vi "ScaleTo16Bit_IQ_raw.vi"(8 "valid in":bool, 9 "factor":u16, 10 "Q":fxp<+/-,18,1>, 11 "I":fxp<+/-,18,1>) -> (0 "valid out":bool, 3 "32bit integer":u32)   [LabVIEW 2025]
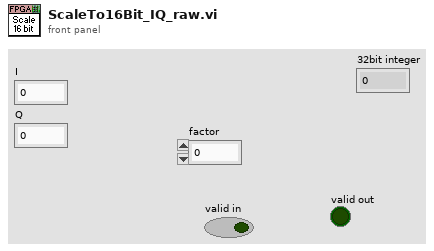
[diagram p1: front panel]
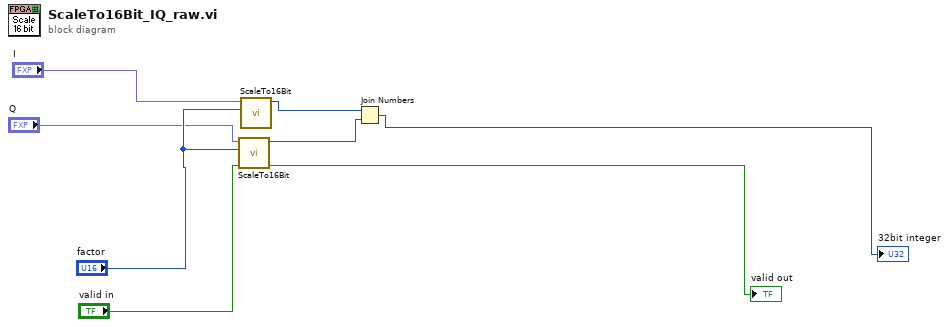
[diagram p0: block diagram]
diagram:
  n1 = call "ScaleTo16Bit.vi"("valid in"="valid in", "factor"="factor", "val"="Q") -> ("valid out"=→"valid out":bool, "16bit integer"=w5:i16)  [unwired: 7 in]
  n2 = call "ScaleTo16Bit.vi"("factor"="factor", "val"="I") -> ("16bit integer"=w6:i16)  [unwired: 8 in, 1 out]
  n3 = Join Numbers(hi=w6, lo=w5) -> ((hi.lo)=→"32bit integer":u32)
